vi "Sending_TestMode_Recipe_Sub_VI.vi"(0 "Socket IP Address":string="192.168.1.100", 1 "Socket Port Numeber":u16=1600, 2 "Receipe Msg ID":i32, 3 "Receipe Message length":i32, 4 "TestAmplitudeLoopC1":i32, 5 "TestAmplitudeLoopC2":i32, 6 "TestPhaseLoopI":i32, 7 "TestPhaseLoopCF":i32, 8 "TestFrequencyHigh":i32, 9 "TestFrequencyLow":i32, 10 "TestAmplitude":i32, 13 "error in (no error)":errorcluster, 14 "Response ID":u8=66) -> (15 "connection ID":refnum<k5>, 16 "Test Mode recipe parameters \nRange validation":string, 17 "error output":errorcluster)   [LabVIEW 2017]
panel:
  out "rest of the binary string":string
  out "String":string=" Success"
  out "bytes written 2":i32
  # "Please find the below information,\n                               \n                                                                Default                 Min                        Max                                                                                         \n \n20KHz System:\n-------------------\nSeekFreqLimitLow                           195000                  195000                     -\nSeekFreqLimitHigh                          205000                       -                         205000\n \n30KHz System:\n-------------------\nSeekFreqLimitLow                           292500                  292500                     -\nSeekFreqLimitHigh                          307500                       -                         307500\n \n40KHz System:\n-------------------\nSeekFreqLimitLow                           395000                  390000                     -\nSeekFreqLimitHigh                          405000                       -                         410000"
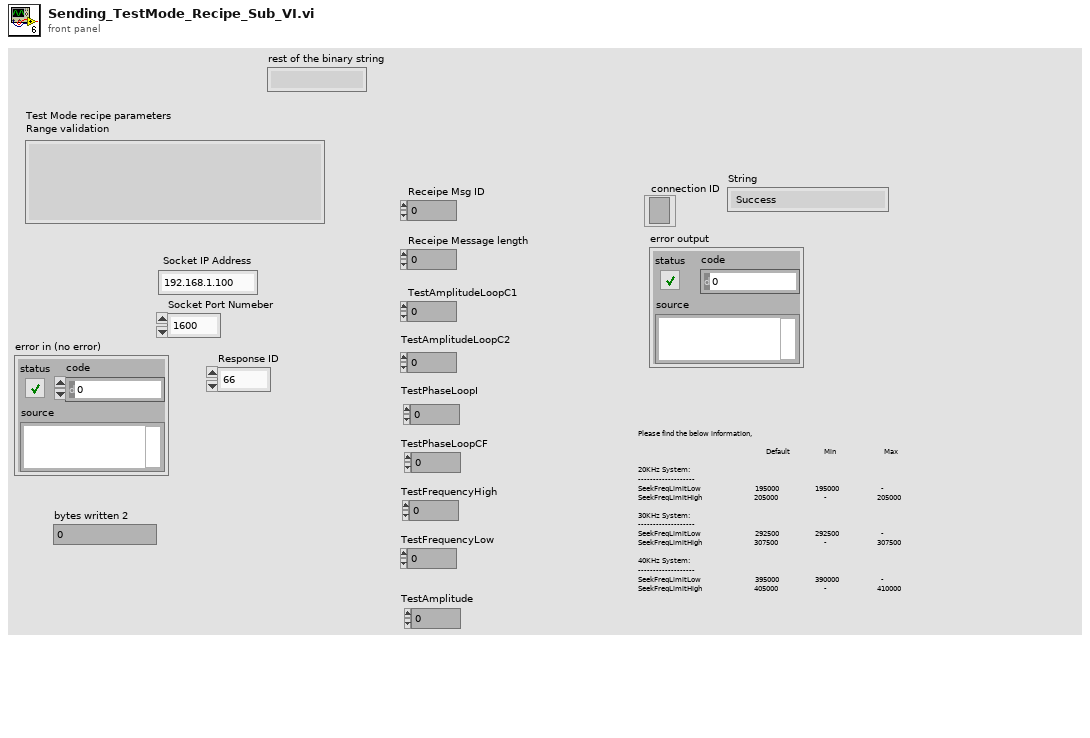
[diagram p1: front panel]
types:
  T1 = enum16{"big-endian, network order", "native, host order", "little-endian"}
  T2 = cluster{"TestAmplitude":i32, "TestFrequencyLow":i32, "TestFrequencyHigh":i32, "TestPhaseLoopCF":i32, "TestPhaseLoopI":i32, "TestAmplitudeLoopC2":i32, "TestAmplitudeLoopC1":i32, "Receipe Message length":i32, "Receipe Msg ID":i32}
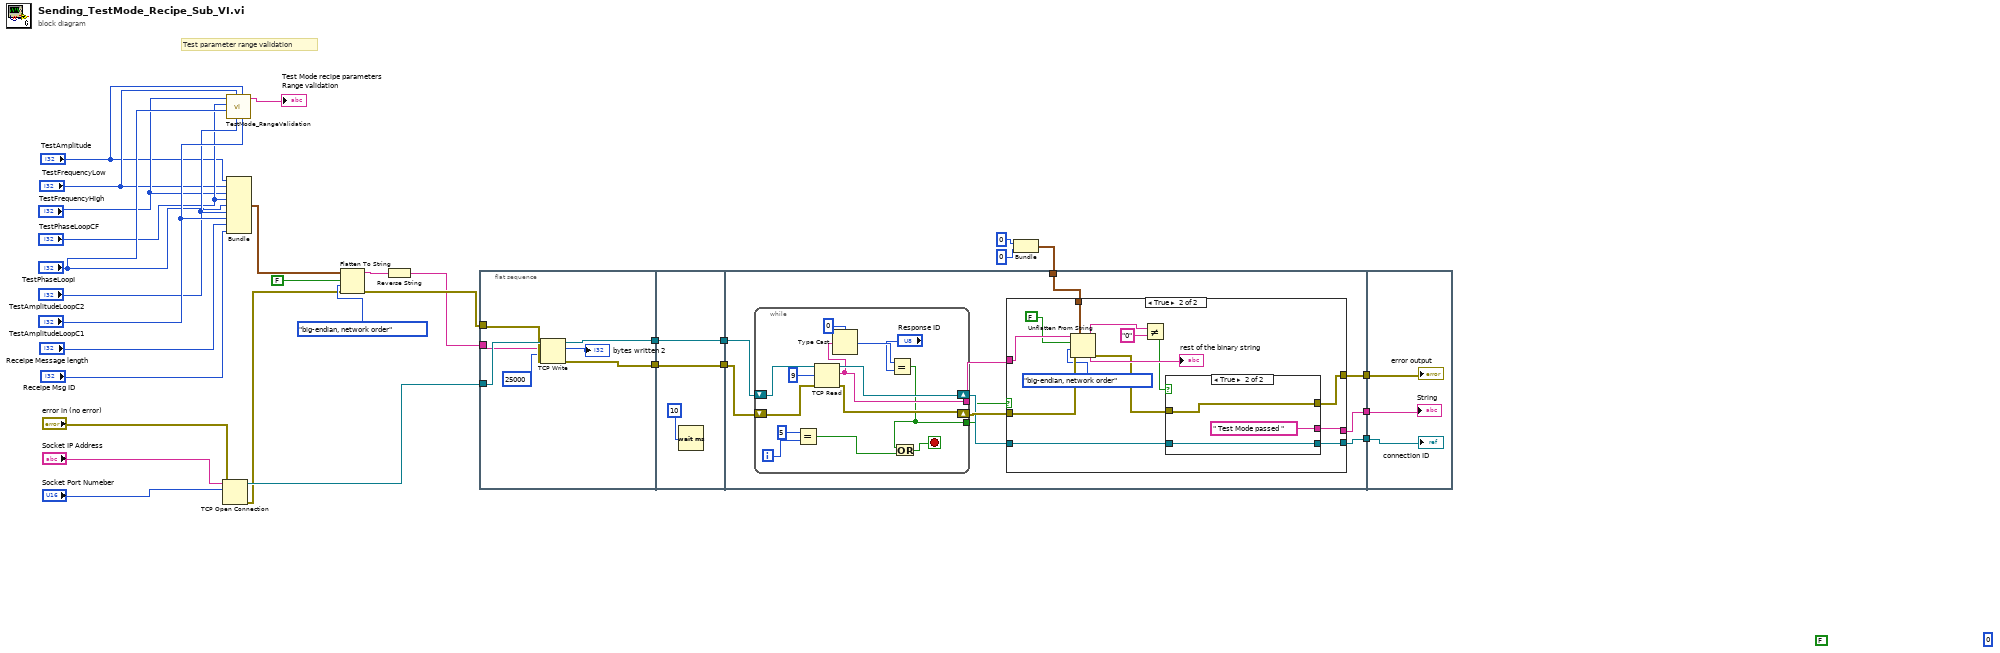
[diagram p0: block diagram]
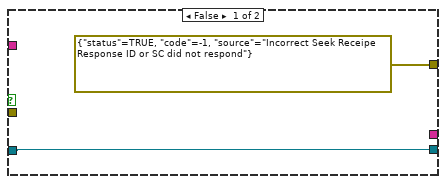
[diagram p2: hidden frame]
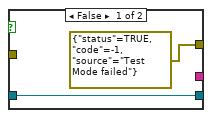
[diagram p3: hidden frame]
diagram:
  (unwired) u8 0
  (unwired) FALSE ("data includes array or string size? (T)")
  # "Test parameter range validation"
  n1 = TCP Open Connection(address="Socket IP Address", remote port or service name="Socket Port Numeber", error in (no error)="error in (no error)") -> (connection ID=w23:refnum<k5>, error out=w22:errorcluster)  [unwired: 2 in]
  n2 = call "TestMode_RangeValidation.vi"("TestAmplitudeLoopC1"="TestAmplitudeLoopC1", "TestAmplitude"="TestAmplitude", "TestAmplitudeLoopC2"="TestAmplitudeLoopC2", "TestFrequencyLow"="TestFrequencyLow", "TestPhaseLoopI"="TestPhaseLoopI", "TestPhaseLoopCF"="TestPhaseLoopCF", "TestFrequencyHigh"="TestFrequencyHigh") -> ("String"=→"Test Mode recipe parameters \nRange validation":string)  [unwired: 4 in]
  n3 = Bundle("TestAmplitude"="TestAmplitude", "TestFrequencyLow"="TestFrequencyLow", "TestFrequencyHigh"="TestFrequencyHigh", "TestPhaseLoopCF"="TestPhaseLoopCF", "TestPhaseLoopI"="TestPhaseLoopI", "TestAmplitudeLoopC2"="TestAmplitudeLoopC2", "TestAmplitudeLoopC1"="TestAmplitudeLoopC1", "Receipe Message length"="Receipe Message length", "Receipe Msg ID"="Receipe Msg ID") -> (w16:T2)  [unwired: 1 in]
  n4 = Flatten To String(anything=w16, prepend array or string size? (T)=FALSE, byte order (0:big-endian, network order)=T1."big-endian, network order", error in (no error)=w22) -> (data string=w20:string, error out=w21:errorcluster)  [unwired: 1 out]
  n5 = Reverse String(1:w20) -> (0:w19:string)
  n6 = flat-sequence {
    tunnel: w23 -> [w36]
    tunnel: w21 -> [w35]
    tunnel: w19 -> [w34]
    tunnel: [w38] -> w31
    tunnel: [w37] -> w30
    tunnel: w31 -> [w41]
    tunnel: w30 -> [w40]
    tunnel: [w41] -> w29
    tunnel: [w40] -> w28
    tunnel: w29 -> [w51]
    tunnel: w28 -> [w50]
    tunnel: w13 -> [w45]
    tunnel: [w44] -> w11
    tunnel: [w43] -> w10
    tunnel: [w42] -> w9
    tunnel: w11 -> [w88]
    tunnel: w10 -> [w87]
    tunnel: w9 -> [w86]
    frame #0 {
      n7 = TCP Write(connection ID=w36, data in=w34, error in (no error)=w35, 9:25000 ("timeout ms (25000)")) -> (connection ID out=w38:refnum<k5>, bytes written=→"bytes written 2":i32, error out=w37:errorcluster)
    }
    frame #1 {
      n8 = Wait (ms)(milliseconds to wait=u32 10) -> ()  [unwired: 1 out]
    }
    frame #2 {
      n9 = while {
        tunnel: [w81] -> w48
        shift-right: [w83] -> w47
        shift-left: w51 -> [w85]
        shift-right: [w77] -> w49
        shift-left: w50 -> [w84]
        tunnel: [w75] -> w46
        i -> [w74]
        stop <- w76 stop-if-true
        n10 = Equal?(x=5, y=w74) -> (x = y?=w72:bool)
        n11 = TCP Read(connection ID=w85, bytes to read=9, error in (no error)=w84) -> (connection ID out=w83:refnum<k5>, data out=w81:string, error out=w77:errorcluster)  [unwired: 2 in]
        n12 = Type Cast(type=u8 0, x=w81) -> (*(type *) &x=w79:u8)
        n13 = Equal?(x=w79, y="Response ID") -> (x = y?=w75:bool)
        n14 = Or(x=w75, y=w72) -> (x .or. y?=w76:bool)
      }
      n15 = case shown="True" w46 {
        tunnel: w49 -> [_ w66]
        tunnel: w48 -> [_ w65]
        tunnel: w47 -> [w53 w58]
        tunnel: w45 -> [_ w62]
        tunnel: [w53 w57] -> w44
        tunnel: [errorcluster {"status"=TRUE, "code"=-1, "source"="Incorrect Seek Receipe Response ID or SC did not respond"} ("error constant") w56] -> w43
        tunnel: [_ w55] -> w42
        frame False {
        }
        frame True {
          n16 = Unflatten From String(type=w62, binary string=w65, data includes array or string size? (T)=FALSE, byte order (0:big-endian, network order)=T1."big-endian, network order", error in (no error)=w66) -> (rest of the binary string=w61:string, error out=w54:errorcluster)  [unwired: 1 out]
          "rest of the binary string" <- w61
          n17 = Not Equal?(x=w61, y="0") -> (x != y?=w59:bool)
          n18 = case shown="True" w59 {
            tunnel: [errorcluster {"status"=TRUE, "code"=-1, "source"="Test Mode failed"} ("error constant") w70] -> w56
            tunnel: w58 -> [w67 w69]
            tunnel: [w67 w69] -> w57
            tunnel: [_ " Test Mode passed "] -> w55
            tunnel: w54 -> [_ w70]
            frame False {
            }
            frame True {
            }
          }
        }
      }
    }
    frame #3 {
      "connection ID" <- w88
      "error output" <- w87
      "String" <- w86
    }
  }
  n19 = Bundle(0, 0) -> (w13:cluster{i32, i32})  [unwired: 1 in]
